vi "Extended.ParseSysexMsgI2CReply.vi"(8 "error in":errorcluster, 11 "Sysex Message":u8[](array[numeric]) format="%x") -> (0 "error out":errorcluster, 1 "I2C Register":u64 format="%x", 2 "I2C Address":u8 format="%x", 3 "I2C Data":u16[](array[numeric]) format="%x")   [LabVIEW 2020, in "FirmataClient.lvlib"]
doc: "Builds a message according to the Firmata Protocol Requirements. \n- https://github.com/firmata/protocol\n- https://github.com/firmata/protocol/blob/master/protocol.md"
uses:
  FirmataClient.lvlib
  controls/FirmataProtocolConstants.ctl
panel:
  out "IsValidSysex":bool
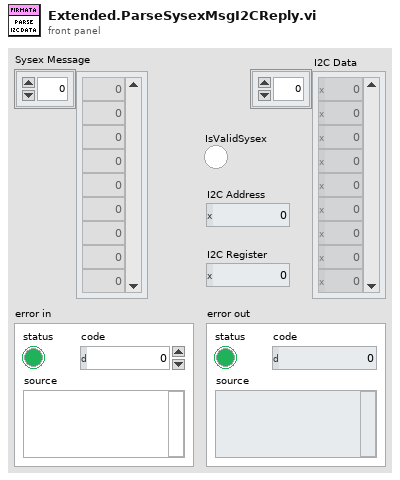
[diagram p1: front panel]
types:
  T1 = typedef "FirmataClient.lvlib/FirmataProtocolConstants.ctl" = u16
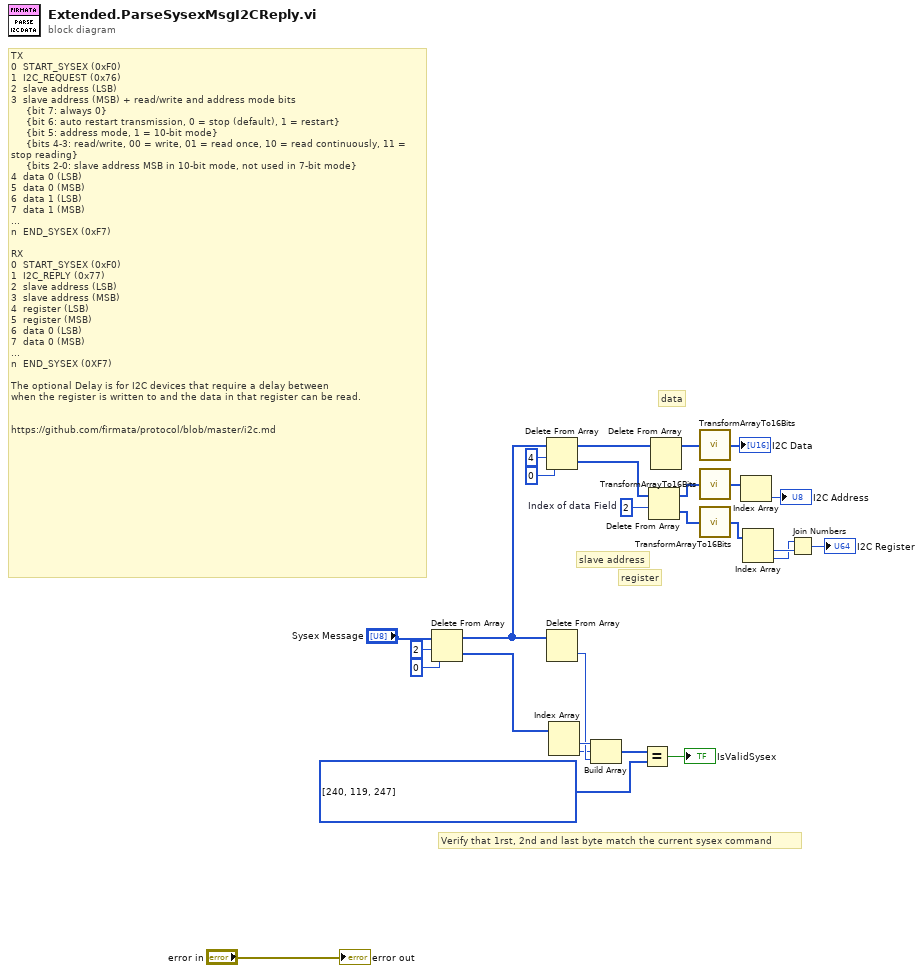
[diagram p0: block diagram]
diagram:
  w21 = T1[] [240, 119, 247] items=["ANALOG_IO_MESSAGE"=224, "DIGITAL_IO_MESSAGE"=144, "REPORT_ANALOG_PIN"=192, "REPORT_DIGITAL_PORT"=208, "START_SYSEX"=240, "END_SYSEX"=247, "SET_PIN_MODE"=244, "SET_DIGITAL_PIN_VALUE"=245, "PROTOCOL_VERSION"=249, "SYSTEM_RESET"=255, "SYSEX.EXTENDED_ID"=0, "SYSEX.RESERVED_USER_COMMANDs"=1, "SYSEX.ANALOG_MAPPING_QUERY"=105, "SYSEX.ANALOG_MAPPING_RESPONSE"=106, "SYSEX.CAPABILITY_QUERY"=107, "SYSEX.CAPABILITY_RESPONSE"=108, "SYSEX.PIN_STATE_QUERY"=109, "SYSEX.PIN_STATE_RESPONSE"=110, "SYSEX.REPORT_FIRMWARE"=121, "SYSEX.EXTENDED_ANALOG"=111, "SYSEX.STRING_DATA"=113, "SYSEX.REALTIME"=127, "SYSEX.NON_REALTIME"=126, "SYSEX.SAMPLING_INTERVAL"=122, "FEATURES.SYSEX.I2C_READ_WRITE"=118, "FEATURES.SYSEX.I2C_REPLY"=119, "FEATURES.SYSEX.I2C_CONFIG"=120]
  w14 = 2  # Index of data Field
  # "register"
  # "slave address"
  # "data"
  # "Verify that 1rst, 2nd and last byte match the current sysex command"
  # "TX\n0  START_SYSEX (0xF0)\n1  I2C_REQUEST (0x76)\n2  slave address (LSB)\n3  slave address (MSB) + read/write and address mode bits\n     {bit 7: always 0}\n     {bit 6: auto restart transmission, 0 = stop (default), 1 = restart}\n     {bit 5: address mode, 1 = 10-bit mode}\n     {bits 4-3: read/write, 00 = write, 01 = read once, 10 = read continuously, 11 = stop reading}\n     {bits 2-0: slave address MSB in 10-bit mode, not used in 7-bit mode}\n4  data 0 (LSB)\n5  data 0 (MSB)\n6  data 1 (LSB)\n7  data 1 (MSB)\n...\nn  END_SYSEX (0xF7)\n\nRX\n0  START_SYSEX (0xF0)\n1  I2C_REPLY (0x77)\n2  slave address (LSB)\n3  slave address (MSB)\n4  register (LSB)\n5  register (MSB)\n6  data 0 (LSB)\n7  data 0 (MSB)\n...\nn  END_SYSEX (0XF7)\n\nThe optional Delay is for I2C devices that require a delay between \nwhen the register is written to and the data in that register can be read.\n\n\nhttps://github.com/firmata/protocol/blob/master/i2c.md"
  n1 = Delete From Array(array="Sysex Message", length=2, index=0) -> (deleted portion=w16:u8[], array with subset deleted=w15:u8[])
  n2 = Delete From Array(array=w15, length=4, index=0) -> (deleted portion=w19:u8[], array with subset deleted=w2:u8[])
  n3 = Delete From Array(array=w15) -> (deleted portion=w25:u8)  [unwired: 2 in, 1 out]
  n4 = Index Array(array=w16) -> (element #1=w26:u8, element #2=w24:u8)  [unwired: 2 in]
  n5 = Build Array(w26, w24, w25) -> (w23:u8[])
  n6 = Equal?(x=w23, y=w21) -> (x = y?=→"IsValidSysex":bool)
  n7 = Delete From Array(array=w19, length=w14) -> (deleted portion=w12:u8[], array with subset deleted=w13:u8[])  [unwired: 1 in]
  n8 = Delete From Array(array=w2) -> (array with subset deleted=w1:u8[])  [unwired: 2 in, 1 out]
  n9 = call "TransformArrayTo16Bits.vi"("Bytes In"=w1) -> ("Byte Out"=→"I2C Data":u16[])
  n10 = call "TransformArrayTo16Bits.vi"("Bytes In"=w13) -> ("Byte Out"=w10:u16[])
  n11 = call "TransformArrayTo16Bits.vi"("Bytes In"=w12) -> ("Byte Out"=w8:u16[])
  n12 = Index Array(array=w10) -> (element=→"I2C Address":u16)  [unwired: 1 in]
  n13 = Index Array(array=w8) -> (element #1=w7:u16, element #2=w6:u16)  [unwired: 2 in]
  n14 = Join Numbers(hi=w6, lo=w7) -> ((hi.lo)=→"I2C Register":u32)
  "error out" <- "error in"
